vi "Alicat_MCQ_stable.vi"() -> ()   [LabVIEW 2023]
panel:
  in  "stop":bool
  out "Measurement Data":T1
  # "Totalizer Timer"
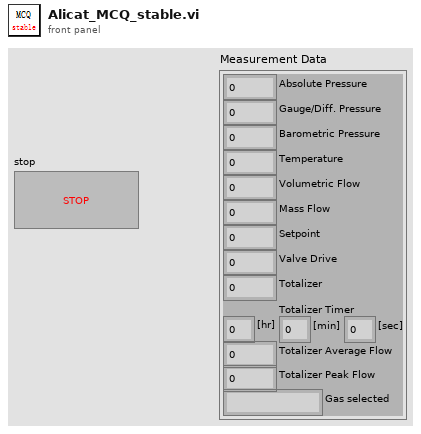
[diagram p1: front panel]
types:
  T1 = cluster{"Absolute Pressure":dbl, "Gauge/Diff. Pressure":dbl, "Barometric Pressure":dbl, "Temperature":dbl, "Volumetric Flow":dbl, "Mass Flow":dbl, "Setpoint":dbl, "Valve Drive":dbl, "Totalizer":dbl, "[hr]":dbl, "[min]":dbl, "[sec]":dbl, "Totalizer Average Flow":dbl, "Totalizer Peak Flow":dbl, "Gas selected":string}
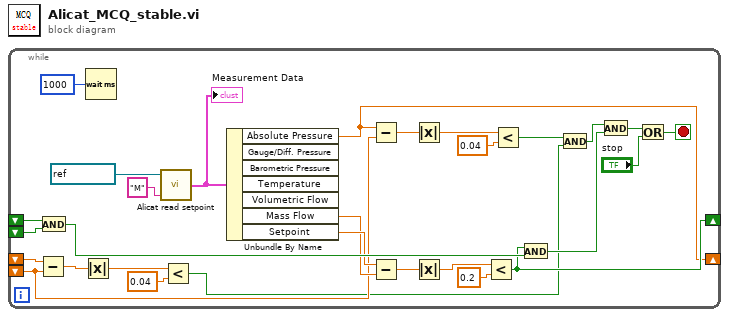
[diagram p0: block diagram]
diagram:
  n1 = while {
    shift-right: [w8] -> _
    shift-left: _ -> [w3]
    shift-left: _ -> [w2]
    shift-right: [w12] -> _
    shift-left: _ -> [w23]
    shift-left: _ -> [w22]
    stop <- w24 stop-if-true
    n2 = Subtract(x=w3, y=w2) -> (x-y=w6:dbl)
    n3 = And(x=w23, y=w22) -> (x .and. y?=w21:bool)
    n4 = Absolute Value(x=w6) -> (abs(x)=w5:dbl)
    n5 = Wait (ms)(milliseconds to wait=u32 1000) -> ()  [unwired: 1 out]
    n6 = call "Alicat read setpoint.vi"("Unit ID"="M", "ALICAT COM Port"=refnum<visa-resource-name> "COM5") -> ("Measurement Data"=w27:T1)  [unwired: 3 in]
    "Measurement Data" <- w27
    n7 = Less?(x=w5, y=0.04) -> (x < y?=w1:bool)
    n8 = Unbundle By Name(w27) -> ("Absolute Pressure"=w8:dbl, "Mass Flow"=w16:dbl, "Setpoint"=w17:dbl)  [unwired: 4 out]
    n9 = Subtract(x=w8, y=w2) -> (x-y=w9:dbl)
    n10 = Subtract(x=w17, y=w16) -> (x-y=w15:dbl)
    n11 = Absolute Value(x=w9) -> (abs(x)=w10:dbl)
    n12 = Absolute Value(x=w15) -> (abs(x)=w14:dbl)
    n13 = Less?(x=w14, y=0.2) -> (x < y?=w12:bool)
    n14 = Less?(x=w10, y=0.04) -> (x < y?=w7:bool)
    n15 = And(x=w12, y=w21) -> (x .and. y?=w20:bool)
    n16 = And(x=w7, y=w1) -> (x .and. y?=w19:bool)
    n17 = And(x=w19, y=w20) -> (x .and. y?=w18:bool)
    n18 = Or(x=w18, y="stop") -> (x .or. y?=w24:bool)
  }
